vi "Set Image Attributes.vi"(10 "AutoBalance":bool, 11 "Refnum in":T1) -> (0 "error out":errorcluster, 3 "Refnum out":T1)   [LabVIEW 2015]
uses:
  <vilib>/userdefined/High Color/IMAQdx.ctl
  <resource>/objmgr/imaqdx.rc
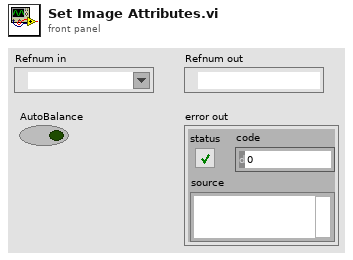
[diagram p1: front panel]
types:
  T1 = typedef "IMAQdx.ctl" = refnum<k21>
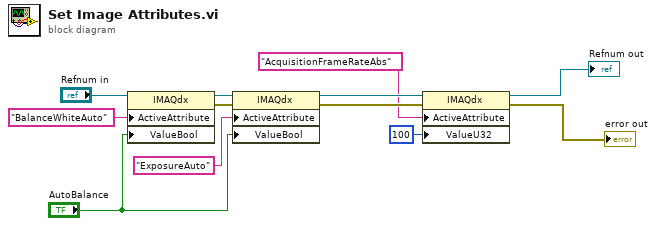
[diagram p0: block diagram]
diagram:
  n1 = property class="IMAQdx"(reference="Refnum in", "ActiveAttribute"="BalanceWhiteAuto", "ValueBool"="AutoBalance") -> (reference out=w10:T1, error out=w11:errorcluster)  [unwired: 1 in]
  n2 = property class="IMAQdx"(reference=w10, error in=w11, "ActiveAttribute"="ExposureAuto", "ValueBool"="AutoBalance") -> (reference out=w6:T1, error out=w4:errorcluster)
  n3 = property class="IMAQdx"(reference=w6, error in=w4, "ActiveAttribute"="AcquisitionFrameRateAbs", "ValueU32"=u32 100) -> (reference out=→"Refnum out":T1, error out=→"error out":errorcluster)
